vi "InitializeSettings.Do.vi"(8 "error in (no error)":errorcluster, 10 "State Variables":T9, 11 "gRPC Request":T1) -> (0 "error out":errorcluster, 2 "State Variables out":T9, 3 "gRPC Response":T6)   [LabVIEW 2025, in "bus_monitor_server_do.lvlib"]
doc: "Initialize the XNET Outgoing Session.\nCreate filter DVR for Incoming Session."
uses:
  bus_monitor_server_do.lvlib
  bus_monitor_server/RPC Messages/ni_bus_monitor_api_InitializeSettingsReply.ctl
  bus_monitor_server/bus_monitor_server.lvlib
  <resource>/objmgr/xnet.rc
  bus_monitor_server/RPC Messages/ni_bus_monitor_api_Session.ctl
  <vilib>/xnet/xnet.llb/XNET Create Session (Frame Output Stream).vi
  bus_monitor_server/RPC Messages/ni_bus_monitor_api_ErrorInfo.ctl
  <vilib>/numeric/Random Number (Range) U64.vi
  bus_monitor_server/RPC Messages/ni_bus_monitor_api_FilterInfo.ctl
  bus_monitor_server/RPC Messages/ni_bus_monitor_api_ConnectSettings.ctl
  Types/XNET.InitialSettings.ctl
  Types/StreamProcess.VIRef.ctl
  Types/StreamProcess.Refs.ctl
  Types/MainProcess.StateVariables.ctl
  bus_monitor_server/RPC Messages/ni_bus_monitor_api_InitializeSettingsRequest.ctl
  bus_monitor_server/RPC Messages/ni_bus_monitor_api_FdIsoMode.ctl
  bus_monitor_server/RPC Messages/ni_bus_monitor_api_Termination.ctl
  bus_monitor_server/RPC Messages/ni_bus_monitor_api_CanMode.ctl
  bus_monitor_server/RPC Messages/ni_bus_monitor_api_FrameFilter.ctl
  bus_monitor_server/RPC Messages/ni_bus_monitor_api_DirectionFilter.ctl
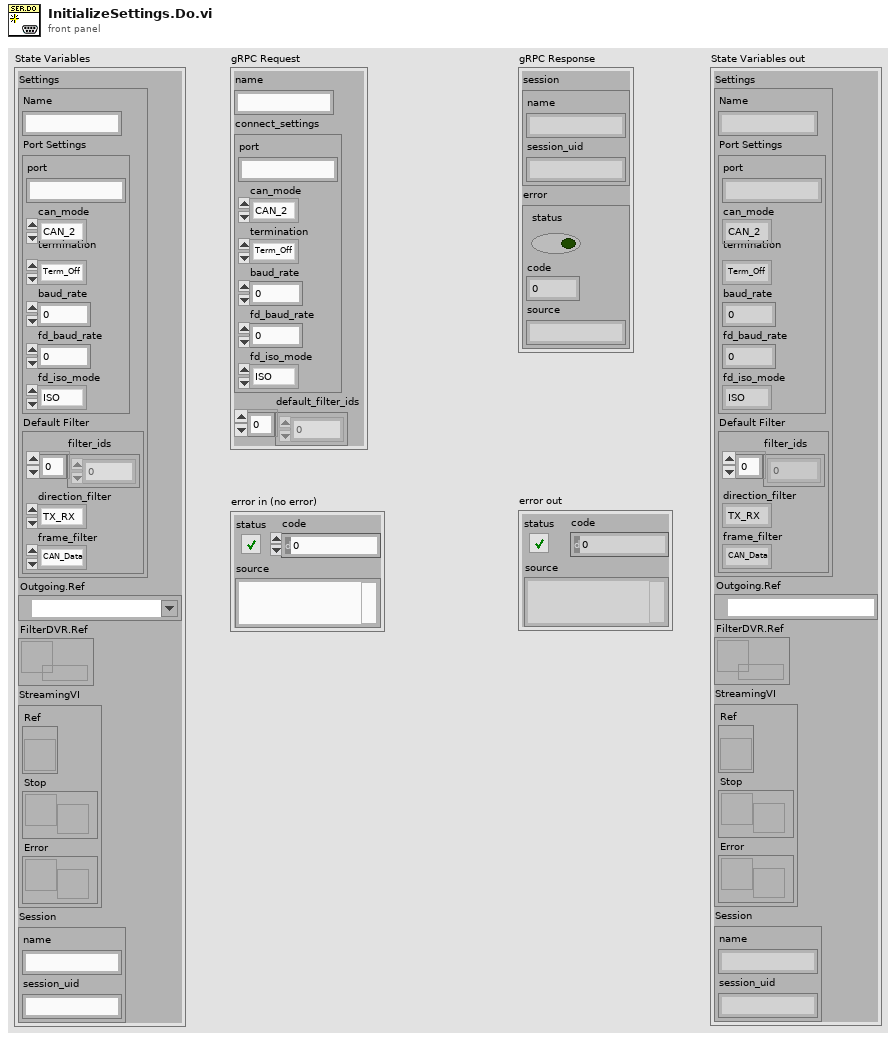
[diagram p1: front panel]
types:
  T1 = typedef "bus_monitor_server.lvlib/ni_bus_monitor_api_InitializeSettingsRequest.ctl" = cluster{"name":string, "connect_settings":T2, "default_filter_ids":u32[]}
  T2 = typedef "bus_monitor_server.lvlib/ni_bus_monitor_api_ConnectSettings.ctl" = cluster{"port":string, "can_mode":T3, "termination":T4, "baud_rate":u64, "fd_baud_rate":u64, "fd_iso_mode":T5}
  T3 = typedef "bus_monitor_server.lvlib/ni_bus_monitor_api_CanMode.ctl" = enum32{"CAN_2", "CAN_FD", "CAN_FD_BRS"}
  T4 = typedef "bus_monitor_server.lvlib/ni_bus_monitor_api_Termination.ctl" = enum32{"Term_Off", "Term_On"}
  T5 = typedef "bus_monitor_server.lvlib/ni_bus_monitor_api_FdIsoMode.ctl" = enum32{"ISO", "Non_ISO", "ISO_Legacy"}
  T6 = typedef "bus_monitor_server.lvlib/ni_bus_monitor_api_InitializeSettingsReply.ctl" = cluster{"session":T7, "error":T8}
  T7 = typedef "bus_monitor_server.lvlib/ni_bus_monitor_api_Session.ctl" = cluster{"name":string, "session_uid":string}
  T8 = typedef "bus_monitor_server.lvlib/ni_bus_monitor_api_ErrorInfo.ctl" = errorcluster
  T9 = typedef "bus_monitor_server_do.lvlib/MainProcess.StateVariables.ctl" = cluster{"Settings":T10, "Outgoing.Ref":refnum<k21>, "FilterDVR.Ref":refnum<data-value>, "StreamingVI":T14, "Session":T7}
  T10 = typedef "bus_monitor_server_do.lvlib/XNET.InitialSettings.ctl" = cluster{"Name":string, "Port Settings":T2, "Default Filter":T11}
  T11 = typedef "bus_monitor_server.lvlib/ni_bus_monitor_api_FilterInfo.ctl" = cluster{"filter_ids":u32[], "direction_filter":T12, "frame_filter":T13}
  T12 = typedef "bus_monitor_server.lvlib/ni_bus_monitor_api_DirectionFilter.ctl" = enum32{"TX_RX", "RX", "TX"}
  T13 = typedef "bus_monitor_server.lvlib/ni_bus_monitor_api_FrameFilter.ctl" = enum32{"CAN_Data", "CAN_Remote", "CAN_Bus_Error", "CAN_2_Data", "CAN_FD_Data", "CAN_FD_BRS_Data", "J1939_Data", "Delay", "Log_Trigger", "Start_Trigger", "All"}
  T14 = typedef "bus_monitor_server_do.lvlib/StreamProcess.Refs.ctl" = cluster{"Ref":T15, "Stop":refnum<notifier>, "Error":refnum<notifier>}
  T15 = typedef "bus_monitor_server_do.lvlib/StreamProcess.VIRef.ctl" = refnum<vi>
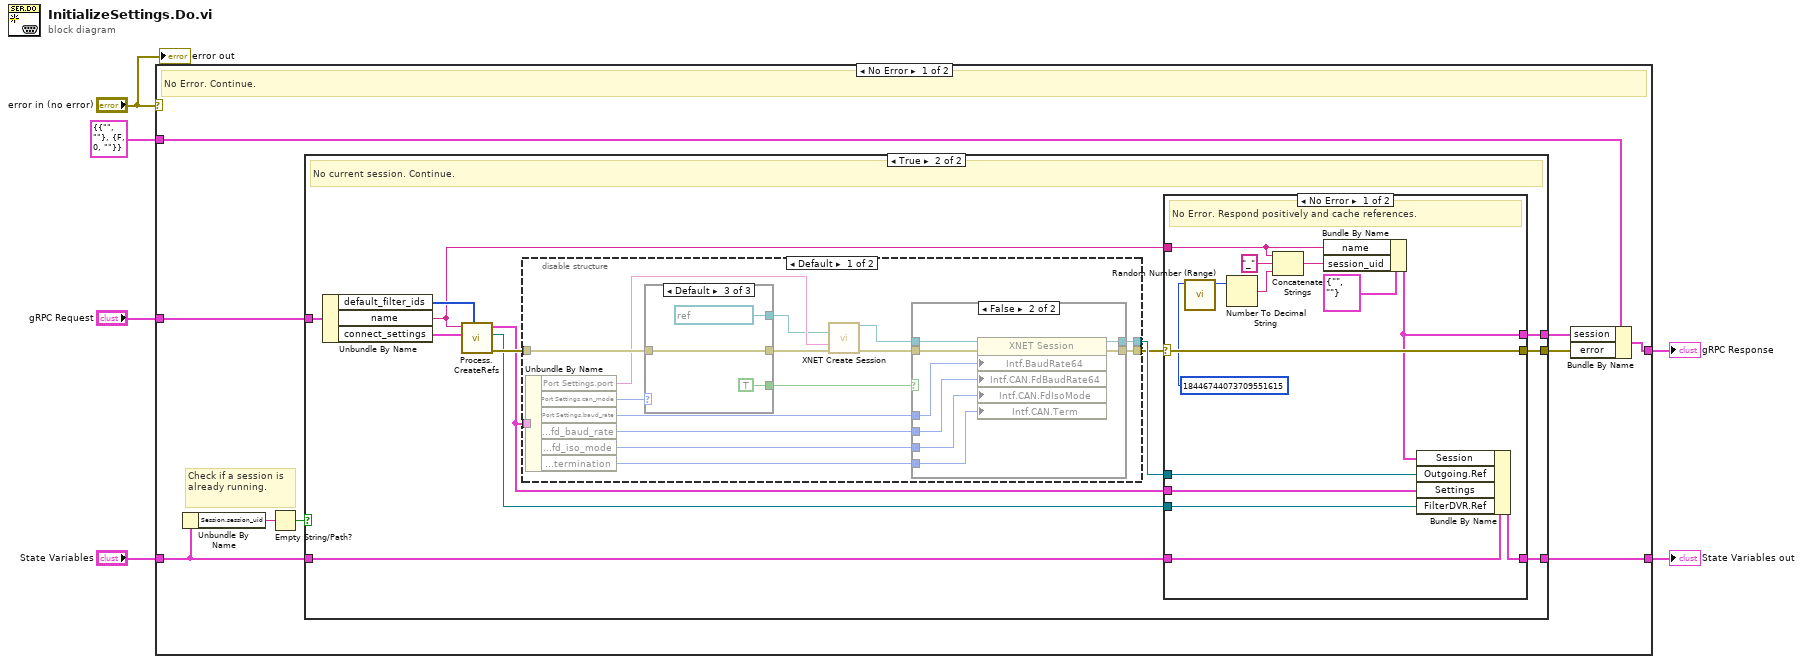
[diagram p0: block diagram]
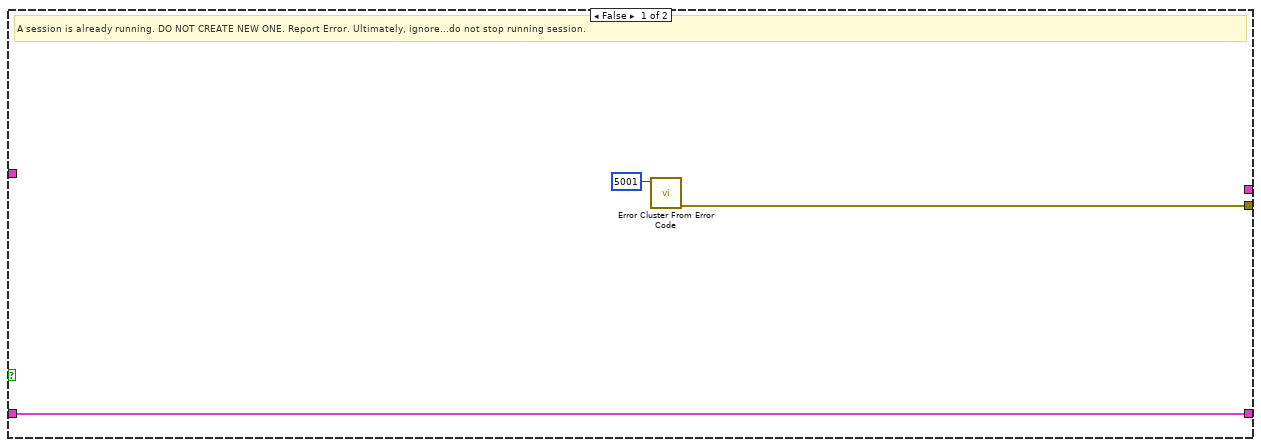
[diagram p2: hidden frame]
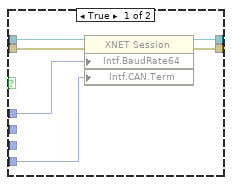
[diagram p3: hidden frame]
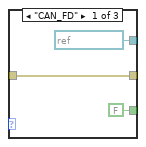
[diagram p4: hidden frame]
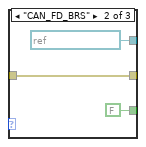
[diagram p5: hidden frame]
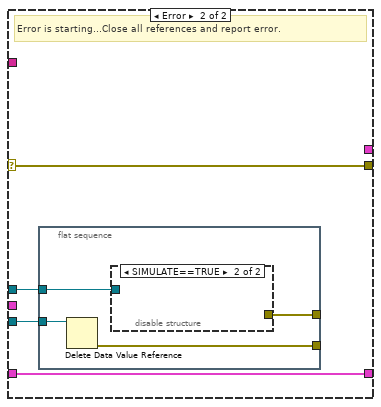
[diagram p7: hidden frame]
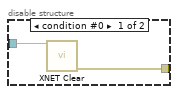
[diagram p8: hidden frame]
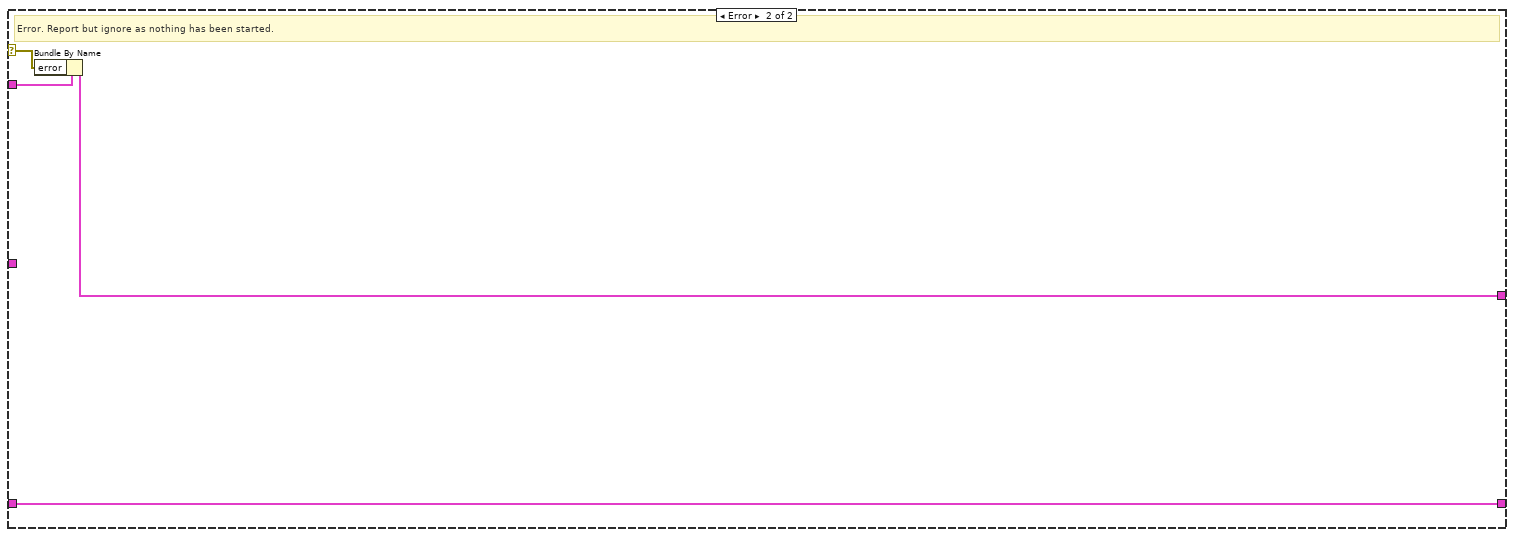
[diagram p9: hidden frame]
diagram:
  n1 = case shown="No Error" "error in (no error)" {
    selector: "error in (no error)" -> [_ w96]
    tunnel: "State Variables" -> [w14 w98]
    tunnel: [w13 w98] -> w5
    tunnel: [w10 w95] -> w4
    tunnel: "gRPC Request" -> [w9 _]
    tunnel: T6 {"session"={"name"="", "session_uid"=""}, "error"={"status"=FALSE, "code"=0, "source"=""}} ("Message Data") -> [w8 w97]
    frame No Error {
      # "Check if a session is already running."
      # "No Error. Continue."
      n2 = Unbundle By Name(w14) -> ("Session.session_uid"=w15:string)
      n3 = Empty String/Path?(string/path=w15) -> (empty?=w12:bool)
      n4 = case shown="True" w12 {
        tunnel: w9 -> [_ w31]
        tunnel: [w18 w24] -> w13
        tunnel: [w17 w21] -> w11
        tunnel: w14 -> [w18 w28]
        tunnel: [_ w20] -> w7
        frame False {
          # "A session is already running. DO NOT CREATE NEW ONE. Report Error. Ultimately, ignore...do not stop running session."
          n5 = call <vilib>:"Error Cluster From Error Code.vi"("error code (0)"=5001) -> ("error out"=w17:errorcluster)  [unwired: 8 in]
        }
        frame True {
          # "No current session. Continue."
          n6 = Unbundle By Name(w31) -> ("default_filter_ids"=w23:u32[], "name"=w19:string, "connect_settings"=w30:T2)
          n7 = call "Process.CreateRefs.vi"("Default IDs"=w23, "Port Settings"=w30, "Name"=w19) -> ("error out"=w29:errorcluster, "FilterDVR.Ref"=w26:refnum<data-value>, "Initial Settings"=w27:T10)  [unwired: 6 in]
          n8 = disable-structure shown="Default" {
            disable-tunnel: w29 -> [w46 w70]
            disable-tunnel: w27 -> [w34 _]
            disable-tunnel: [w33 _] -> w25
            disable-tunnel: [w32 w70] -> w22
            frame condition #0 {
              n9 = Unbundle By Name(w34) -> ("Port Settings.port"=w45:string, "Port Settings.can_mode"=w42:T3, "Port Settings.baud_rate"=w43:u64, "Port Settings.fd_baud_rate"=w44:u64, "Port Settings.fd_iso_mode"=w41:T5, "Port Settings.termination"=w37:T4)
              n10 = case shown="Default" w42 {
                tunnel: [refnum<k21> ":can_fd:" ("cluster (:memory:)") refnum<k21> ":can_fd_brs:" ("cluster (:memory:)") refnum<k21> ":memory:" ("cluster (:memory:)")] -> w38
                tunnel: w46 -> [w61 w64 w67]
                tunnel: [w61 w64 w67] -> w39
                tunnel: [FALSE FALSE TRUE] -> w40
                frame "CAN_FD" {
                }
                frame "CAN_FD_BRS" {
                }
                frame Default {
                }
              }
              n11 = call-poly <vilib>:"XNET Create Session.vi"("cluster (:memory:)"=w38, "interface"=w45, "error in (no error)"=w39) -> ("session out"=w35:refnum<k21>, "error out"=w36:errorcluster)  [unwired: 11 out]
              n12 = case shown="False" w40 {
                tunnel: w35 -> [w52 w60]
                tunnel: [w51 w59] -> w33
                tunnel: w36 -> [w50 w58]
                tunnel: [w49 w57] -> w32
                tunnel: w37 -> [w47 w56]
                tunnel: w43 -> [w48 w55]
                tunnel: w41 -> [_ w54]
                tunnel: w44 -> [_ w53]
                frame True {
                  n13 = property class="XNET Session"(reference=w52, error in=w50, "Intf.BaudRate64"=w48, "Intf.CAN.Term"=w47) -> (reference out=w51:refnum<k21>, error out=w49:errorcluster)
                }
                frame False {
                  n14 = property class="XNET Session"(reference=w60, error in=w58, "Intf.BaudRate64"=w55, "Intf.CAN.FdBaudRate64"=w53, "Intf.CAN.FdIsoMode"=w54, "Intf.CAN.Term"=w56) -> (reference out=w59:refnum<k21>, error out=w57:errorcluster)
                }
              }
            }
            frame condition #1 (active) {
            }
          }
          n15 = case shown="No Error" w22 {
            selector: w22 -> [w79 w88]
            tunnel: w28 -> [w84 w85]
            tunnel: w27 -> [w83 _]
            tunnel: w26 -> [w82 w86]
            tunnel: w25 -> [w81 w87]
            tunnel: [w80 w85] -> w24
            tunnel: [w79 w88] -> w21
            tunnel: [w72 _] -> w20
            tunnel: w19 -> [w75 _]
            frame No Error {
              # "No Error. Respond positively and cache references."
              n16 = call-poly <vilib>:"Random Number (Range).vi"("upper bound (100)"=u64 18446744073709551615) -> ("number"=w76:u64)  [unwired: 10 in]
              n17 = Number To Decimal String(number=w76) -> (decimal integer string=w74:string)  [unwired: 1 in]
              n18 = Concatenate Strings(w75, "_" ("string"), w74) -> (w77:string)
              n19 = Bundle By Name(cluster=T7 {"name"="", "session_uid"=""} ("session"), "name"=w75, "session_uid"=w77) -> (w72:T7)
              n20 = Bundle By Name(cluster=w84, "Session"=w72, "Outgoing.Ref"=w81, "Settings"=w83, "FilterDVR.Ref"=w82) -> (w80:T9)
            }
            frame Error {
              # "Error is starting...Close all references and report error."
              n21 = flat-sequence {
                tunnel: w87 -> [w92]
                tunnel: w86 -> [w91]
                tunnel: [w90] -> _
                tunnel: [w89] -> _
                frame #0 {
                  n22 = Delete Data Value Reference(data value reference=w91) -> (error out=w89:errorcluster)  [unwired: 1 in, 1 out]
                  n23 = disable-structure shown="SIMULATE==TRUE" {
                    disable-tunnel: w92 -> [w94 _]
                    disable-tunnel: [w93 _] -> w90
                    frame condition #0 {
                      n24 = call <vilib>:"XNET Clear.vi"("session in"=w94) -> ("error out"=w93:errorcluster)  [unwired: 14 in]
                    }
                    frame condition #1 (active) {
                    }
                  }
                }
              }
            }
          }
        }
      }
      n25 = Bundle By Name(cluster=w8, "session"=w7, "error"=w11) -> (w10:T6)
    }
    frame Error {
      # "Error. Report but ignore as nothing has been started."
      n26 = Bundle By Name(cluster=w97, "error"=w96) -> (w95:T6)
    }
  }
  "State Variables out" <- w5
  "gRPC Response" <- w4
  "error out" <- "error in (no error)"
